vi "Replace Item.vi"(8 "error in (no error)":errorcluster, 10 "Tag":refnum<class "Tree Tag Class.lvclass">, 11 "Tree_LVOOP in":refnum<class "Tree Class.lvclass">) -> (0 "error out":errorcluster, 3 "Tree_LVOOP out":refnum<class "Tree Class.lvclass">)   [LabVIEW 2012, in "Tree Tools.lvlib" / "Tree Class.lvclass"]
uses:
  Tree Class.lvclass
  Tree Tag Class/Tree Tag Class.lvclass
  Tree Class.lvclass/Tree Class.ctl
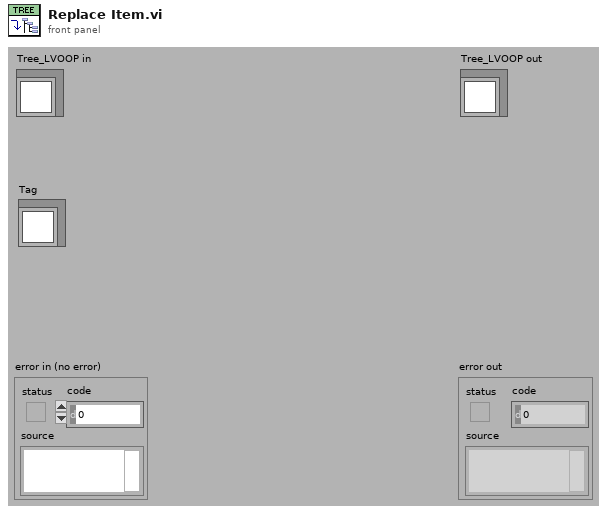
[diagram p1: front panel]
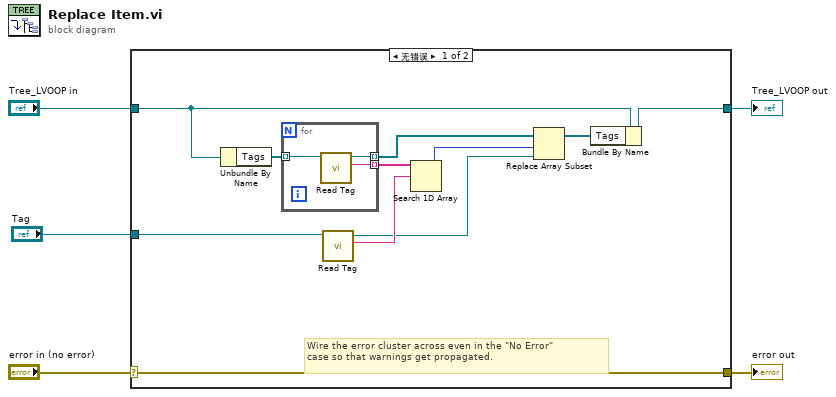
[diagram p0: block diagram]
diagram:
  n1 = case shown="无错误" "error in (no error)" {
    selector: "error in (no error)" -> [w16 w21]
    tunnel: [w16 w21] -> w4
    tunnel: [w10 w20] -> w2
    tunnel: "Tree_LVOOP in" -> [w11 w20]
    tunnel: "Tag" -> [w14 _]
    frame No Error {
      # "Wire the error cluster across even in the \"No Error\"\ncase so that warnings get propagated."
      n2 = Unbundle By Name(w11) -> ("Tags"=w15:refnum<class "Tree Tag Class.lvclass">[])
      n3 = for {
        tunnel: w15 -> [w19] mode=indexing
        tunnel: [w18] -> w13 mode=indexing
        tunnel: [w17] -> w8 mode=indexing
        n4 = call-dynamic "Read Tag.vi"("Tag_LVOOP.lvclass in"=w19) -> ("Tag"=w18:string, "Tag_LVOOP.lvclass out"=w17:refnum<class "Tree Tag Class.lvclass">)  [unwired: 8 in, 1 out]
      }
      n5 = call-dynamic "Read Tag.vi"("Tag_LVOOP.lvclass in"=w14) -> ("Tag"=w12:string, "Tag_LVOOP.lvclass out"=w6:refnum<class "Tree Tag Class.lvclass">)  [unwired: 8 in, 1 out]
      n6 = Search 1D Array(1D array=w13, element=w12) -> (index of element=w7:i32)  [unwired: 1 out]
      n7 = Replace Array Subset(array=w8, new element=w6, index=w7) -> (w9:refnum<class "Tree Tag Class.lvclass">[])
      n8 = Bundle By Name(cluster=w11, "Tags"=w9) -> (w10:refnum<class "Tree Class.lvclass">)
    }
    frame Error {
    }
  }
  "error out" <- w4
  "Tree_LVOOP out" <- w2
